vi "testInvalidRefnum.vi"() -> (0 "error out":errorcluster)   [LabVIEW 2019, in "FactTest.lvlib"]
uses:
  FactTest.lvlib
  Fact/Fact.lvclass
  Assertion/Assertion.lvlib
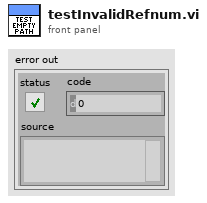
[diagram p1: front panel]
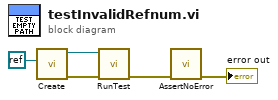
[diagram p0: block diagram]
diagram:
  n1 = call "Create.vi"("VI Refnum"=refnum<k0> refnum) -> ("error out"=w4:errorcluster, "Fact"=w5:refnum<class "Fact.lvclass">)  [unwired: 9 in]
  n2 = call-dynamic "RunTest.vi"("error in (no error)"=w4, "Fact in"=w5) -> ("error out"=w3:errorcluster)  [unwired: 8 in, 1 out]
  n3 = call "AssertNoError.vi"("error in (no error)"=w3) -> ("error out"=→"error out":errorcluster)  [unwired: 10 in]
